vi "TcA01-003_ObjectCreationAndDestructionOfMultipleClasses.vi"(1 "Input buffer":T3="1", 3 "Invocation info":T2, 5 "error in (no error)":errorcluster, 6 "Add log to result?":bool) -> (16 "Test Data":T1 {"Numeric Measurement" format="%.2f"}, 19 "error out":errorcluster)   [LabVIEW 2009]
doc: "Test case template."
uses:
  Shared/Support_InputBuffer.ctl
  Shared/Support_InvocationInfo.ctl
  Shared/Support_TestData.ctl
  TestClasses/G#SubClass2_class/G#SubClass2.lvclass
  TestClasses/G#SubClass1_class/G#SubClass1.lvclass
  TestClasses/G#BaseClass2_class/G#BaseClass2.lvclass
  TestClasses/G#BaseClass1_class/G#BaseClass1.lvclass
  <vilib>/addons/_AddQ/G#Object/G#Object.lvclass
panel:
  in  "Test name":string="TcA01-003 Object creation and destruction of multiple classes"
  out "Test result":bool
  out "Result":string
  # "Verify that objects from different classes can be\ncreated and destroy multiple times simultaneously"
  # "Sub test case"
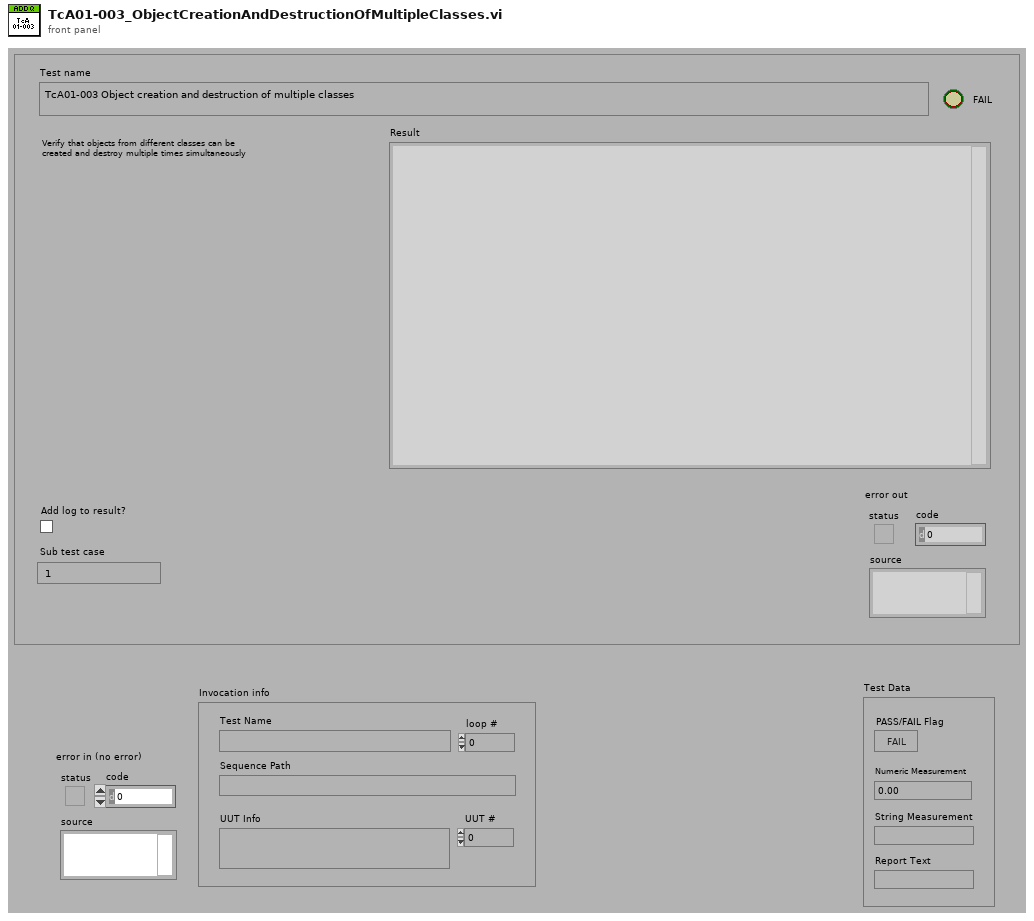
[diagram p1: front panel]
types:
  T1 = typedef "Support_TestData.ctl" = cluster{"PASS/FAIL Flag":bool, "Numeric Measurement":dbl, "String Measurement":string, "Report Text":string}
  T2 = typedef "Support_InvocationInfo.ctl" = cluster{"UUT #":i32, "loop #":i32, "UUT Info":string, "Test Name":string, "Sequence Path":path}
  T3 = typedef "Support_InputBuffer.ctl" = string
  T4 = typedef "Support_ResultType.ctl" = cluster{"Pass":bool, "Comment":string, "MeasurementValue":dbl}
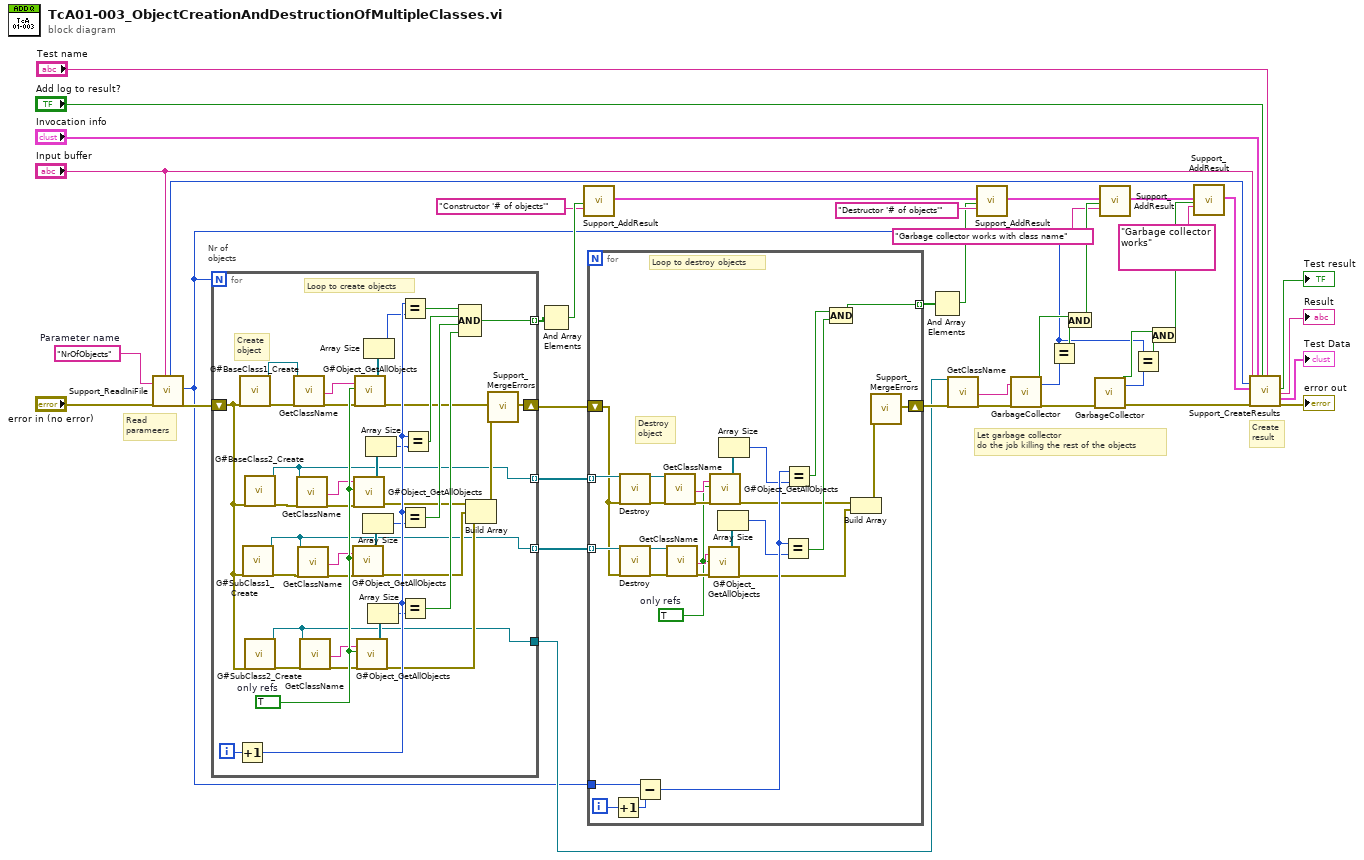
[diagram p0: block diagram]
diagram:
  w36 = "NrOfObjects"  # Parameter name
  # "Let garbage collector\ndo the job killing the rest of the objects"
  # "Read\nparameers"
  # "Create\nresult"
  # "Nr of\nobjects"
  n1 = call "Support_ReadIniFile.vi"("Parameter name"=w36, "error in (no error)"="error in (no error)", "Sub test case"="Input buffer") -> ("Timer start"=w19:u32, "Parameter1 as I32"=w2:i32, "error out"=w34:errorcluster)  [unwired: 9 in, 5 out]
  n2 = for {
    N: w2 -> [_]
    shift-right: [w80] -> w30
    shift-left: w34 -> [w78]
    tunnel: [w72] -> w33 mode=indexing
    tunnel: [w43] -> w11
    tunnel: [w48] -> w22 mode=indexing
    tunnel: [w52] -> w21 mode=indexing
    i -> [w81]
    w59 = TRUE  # only refs
    # "Create\nobject"
    # "Loop to create objects"
    n3 = Increment(x=w81) -> (x+1=w77:i32)
    n4 = call "G#BaseClass1_Create.vi"("error in (no error)"=w78) -> ("reference out"=w56:refnum<class "G#BaseClass1.lvclass">, "error out"=w58:errorcluster)  [unwired: 16 in, 1 out]
    n5 = call "G#SubClass1_Create.vi"("error in (no error)"=w78) -> ("reference out"=w48:refnum<class "G#SubClass1.lvclass">, "error out"=w47:errorcluster)  [unwired: 16 in, 1 out]
    n6 = call "G#BaseClass2_Create.vi"("error in (no error)"=w78) -> ("reference out"=w52:refnum<class "G#BaseClass2.lvclass">, "error out"=w54:errorcluster)  [unwired: 17 in]
    n7 = call "G#SubClass2_Create.vi"("error in (no error)"=w78) -> ("reference out"=w43:refnum<class "G#SubClass2.lvclass">, "error out"=w45:errorcluster)  [unwired: 17 in]
    n8 = call-dynamic "GetClassName.vi"("reference in"=w56, "error in (no error)"=w58) -> ("full class name"=w55:string, "error out"=w57:errorcluster)  [unwired: 13 in, 3 out]
    n9 = call-dynamic "GetClassName.vi"("reference in"=w52, "error in (no error)"=w54) -> ("full class name"=w51:string, "error out"=w53:errorcluster)  [unwired: 13 in, 3 out]
    n10 = call-dynamic "GetClassName.vi"("reference in"=w48, "error in (no error)"=w47) -> ("full class name"=w50:string, "error out"=w46:errorcluster)  [unwired: 13 in, 3 out]
    n11 = call-dynamic "GetClassName.vi"("reference in"=w43, "error in (no error)"=w45) -> ("full class name"=w49:string, "error out"=w44:errorcluster)  [unwired: 13 in, 3 out]
    n12 = call <vilib>:"G#Object_GetAllObjects.vi"("full class name (\"\")"=w50, "only refs (F)"=w59, "error in (no error)"=w46) -> ("all refs"=w61:refnum<class "G#Object.lvclass">[], "error out"=w69:errorcluster)  [unwired: 13 in, 2 out]
    n13 = call <vilib>:"G#Object_GetAllObjects.vi"("full class name (\"\")"=w51, "only refs (F)"=w59, "error in (no error)"=w53) -> ("all refs"=w62:refnum<class "G#Object.lvclass">[], "error out"=w70:errorcluster)  [unwired: 13 in, 2 out]
    n14 = call <vilib>:"G#Object_GetAllObjects.vi"("full class name (\"\")"=w55, "only refs (F)"=w59, "error in (no error)"=w57) -> ("all refs"=w63:refnum<class "G#Object.lvclass">[], "error out"=w71:errorcluster)  [unwired: 13 in, 2 out]
    n15 = call <vilib>:"G#Object_GetAllObjects.vi"("full class name (\"\")"=w49, "only refs (F)"=w59, "error in (no error)"=w44) -> ("all refs"=w60:refnum<class "G#Object.lvclass">[], "error out"=w68:errorcluster)  [unwired: 13 in, 2 out]
    n16 = Array Size(array=w61) -> (size(s)=w65:i32)
    n17 = Array Size(array=w63) -> (size(s)=w67:i32)
    n18 = Array Size(array=w62) -> (size(s)=w66:i32)
    n19 = Array Size(array=w60) -> (size(s)=w64:i32)
    n20 = Equal?(x=w77, y=w67) -> (x = y?=w76:bool)
    n21 = Equal?(x=w77, y=w65) -> (x = y?=w74:bool)
    n22 = Equal?(x=w77, y=w64) -> (x = y?=w73:bool)
    n23 = Equal?(x=w77, y=w66) -> (x = y?=w75:bool)
    n24 = Compound Arithmetic op=AND(w76, w75, w74, w73) -> (w72:bool)
    n25 = Build Array(w70, w69, w68) -> (w79:errorcluster[])
    n26 = call "Support_MergeErrors.vi"("error in 1"=w71, "Error array"=w79) -> ("error out"=w80:errorcluster)  [unwired: 16 in, 1 out]
  }
  n27 = And Array Elements(Boolean array=w33) -> (logical AND=w32:bool)
  n28 = call "Support_AddResult.vi"("Pass"=w32, "Comment"="Constructor '# of objects'") -> ("Results out"=w23:T4[])  [unwired: 17 in]
  n29 = for {
    shift-right: [w101] -> w15
    shift-left: w30 -> [w103]
    tunnel: [w97] -> w29 mode=indexing
    tunnel: w2 -> [w107]
    tunnel: w22 -> [w104] mode=indexing
    tunnel: w21 -> [w105] mode=indexing
    i -> [w108]
    w82 = TRUE  # only refs
    # "Destroy\nobject"
    # "Loop to destroy objects"
    n30 = Increment(x=w108) -> (x+1=w106:i32)
    n31 = call-dynamic "Destroy.vi"("reference in"=w105, "error in (no error)"=w103) -> ("reference out"=w87:refnum<class "G#BaseClass2.lvclass">, "error out"=w90:errorcluster)  [unwired: 16 in]
    n32 = call-dynamic "Destroy.vi"("reference in"=w104, "error in (no error)"=w103) -> ("reference out"=w88:refnum<class "G#SubClass1.lvclass">, "error out"=w89:errorcluster)  [unwired: 16 in]
    n33 = Subtract(x=w107, y=w106) -> (x-y=w102:i32)
    n34 = call-dynamic "GetClassName.vi"("reference in"=w87, "error in (no error)"=w90) -> ("full class name"=w83:string, "error out"=w86:errorcluster)  [unwired: 13 in, 3 out]
    n35 = call-dynamic "GetClassName.vi"("reference in"=w88, "error in (no error)"=w89) -> ("full class name"=w84:string, "error out"=w85:errorcluster)  [unwired: 13 in, 3 out]
    n36 = call <vilib>:"G#Object_GetAllObjects.vi"("full class name (\"\")"=w84, "only refs (F)"=w82, "error in (no error)"=w85) -> ("all refs"=w95:refnum<class "G#Object.lvclass">[], "error out"=w94:errorcluster)  [unwired: 13 in, 2 out]
    n37 = call <vilib>:"G#Object_GetAllObjects.vi"("full class name (\"\")"=w83, "only refs (F)"=w82, "error in (no error)"=w86) -> ("all refs"=w96:refnum<class "G#Object.lvclass">[], "error out"=w93:errorcluster)  [unwired: 13 in, 2 out]
    n38 = Array Size(array=w95) -> (size(s)=w91:i32)
    n39 = Array Size(array=w96) -> (size(s)=w92:i32)
    n40 = Equal?(x=w102, y=w91) -> (x = y?=w98:bool)
    n41 = Equal?(x=w102, y=w92) -> (x = y?=w99:bool)
    n42 = Compound Arithmetic op=AND(w99, w98) -> (w97:bool)
    n43 = Build Array(w93, w94) -> (w100:errorcluster[])
    n44 = call "Support_MergeErrors.vi"("Error array"=w100) -> ("error out"=w101:errorcluster)  [unwired: 17 in, 1 out]
  }
  n45 = And Array Elements(Boolean array=w29) -> (logical AND=w26:bool)
  n46 = call-dynamic "GetClassName.vi"("reference in"=w11, "error in (no error)"=w15) -> ("full class name"=w12:string, "error out"=w14:errorcluster)  [unwired: 13 in, 3 out]
  n47 = call "Support_AddResult.vi"("Results in"=w23, "Pass"=w26, "Comment"="Destructor '# of objects'") -> ("Results out"=w7:T4[])  [unwired: 16 in]
  n48 = call <vilib>:"GarbageCollector.vi"("full class name"=w12, "error in (no error)"=w14) -> ("OK"=w9:bool, "# of objects killed"=w10:i32, "error out"=w13:errorcluster)  [unwired: 15 in]
  n49 = Equal?(x=w2, y=w10) -> (x = y?=w8:bool)
  n50 = And(x=w9, y=w8) -> (x .and. y?=w5:bool)
  n51 = call <vilib>:"GarbageCollector.vi"("error in (no error)"=w13) -> ("OK"=w18:bool, "# of objects killed"=w3:i32, "error out"=w17:errorcluster)  [unwired: 16 in]
  n52 = call "Support_AddResult.vi"("Results in"=w7, "Pass"=w5, "Comment"="Garbage collector works with class name") -> ("Results out"=w6:T4[])  [unwired: 16 in]
  n53 = Equal?(x=w2, y=w3) -> (x = y?=w1:bool)
  n54 = And(x=w18, y=w1) -> (x .and. y?=w16:bool)
  n55 = call "Support_AddResult.vi"("Results in"=w6, "Pass"=w16, "Comment"="Garbage collector works") -> ("Results out"=w25:T4[])  [unwired: 16 in]
  n56 = call "Support_CreateResults.vi"("Sub test case"="Input buffer", "Timer start"=w19, "Results"=w25, "error in (no error)"=w17, "Invocation info"="Invocation info", "Add log to result?"="Add log to result?", "Test name"="Test name") -> ("Pass/fail flag"=→"Test result":bool, "Result"=→"Result":string, "Test Data"=→"Test Data":T1, "error out"=→"error out":errorcluster)  [unwired: 9 in]
